vi "PhaseShifter demo GUI settings.vi"(11 "Settings":T1={"States"=32, "Timeout (ms)"=250, "Frequency (MHz)"=900.0, "IL spec (dB)"=-2.0, "Lookup table"=path "", "Demo Mode"=enum."Live mode", "Board Loss"=0.3}) -> (3 "Settings 2":T1={"States"=32, "Timeout (ms)"=250, "Frequency (MHz)"=900.0, "IL spec (dB)"=-2.0, "Lookup table"=path "", "Demo Mode"=enum."Live mode", "Board Loss"=0.3}, 4 "Reset FoM calculation 2":bool)   [LabVIEW 2020]
uses:
  PhaseShifter demo settings.ctl
panel:
  in  "Reset FoM calculation":bool
  in  "System Cancel Button":bool
  in  "System OK Button":bool
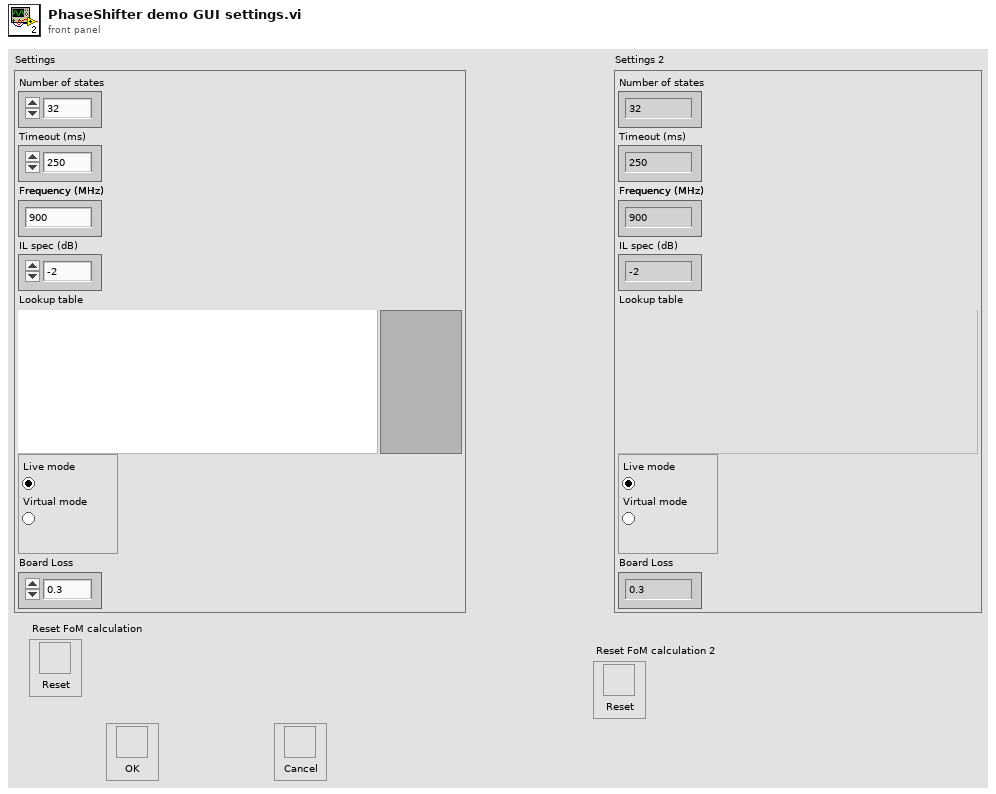
[diagram p1: front panel]
types:
  T1 = typedef "PhaseShifter demo settings.ctl" = cluster{"States":i32, "Timeout (ms)":i32, "Frequency (MHz)":dbl, "IL spec (dB)":dbl, "Lookup table":path, "Demo Mode":enum32{"Live mode", "Virtual mode"}, "Board Loss":dbl}
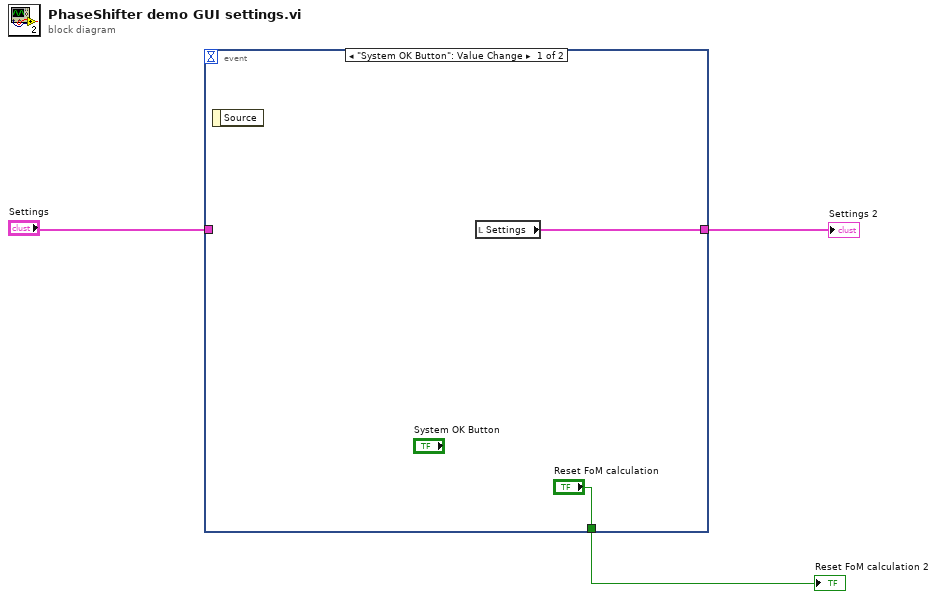
[diagram p0: block diagram]
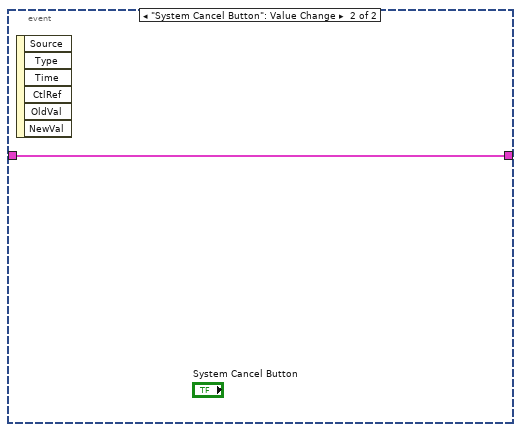
[diagram p2: hidden frame]
diagram:
  n1 = event shown="[0] \"System OK Button\": Value Change" {
    selector: _ -> [_ _]
    dyn-events: _ -> [_ _]
    timeout: _ -> [_ _]
    tunnel: "Settings" -> [_ w6]
    tunnel: [w5 w6] -> w3
    tunnel: ["Reset FoM calculation" _] -> w1
    event "System OK Button": Value Change {
      n2 = event-data() -> ()  [unwired: 1 in, 1 out]
      n3 = local read "Settings"() -> (w5:T1)
    }
    event "System Cancel Button": Value Change {
      n4 = event-data() -> ()  [unwired: 1 in, 6 out]
    }
  }
  "Settings 2" <- w3
  "Reset FoM calculation 2" <- w1
